vi "Open&Close Door Record.vi"(8 "error in (no error)":errorcluster, 11 "Para":T2={"url"="http://dev.watersystem.com.cn:36091", "AccessToken"="data&auXnb5fsZ6235te50ySpHm7Nhv4", "mn"="admin", "isOpenDoor"=FALSE}) -> (0 "error out":errorcluster, 3 "response":T1)   [LabVIEW 2016, in "opSignIn.lvlib"]
uses:
  <vilib>/httpClient/POSTBuffer.vi
  opSignIn.lvlib
  <vilib>/httpClient/LabVIEWHTTPClient.lvlib
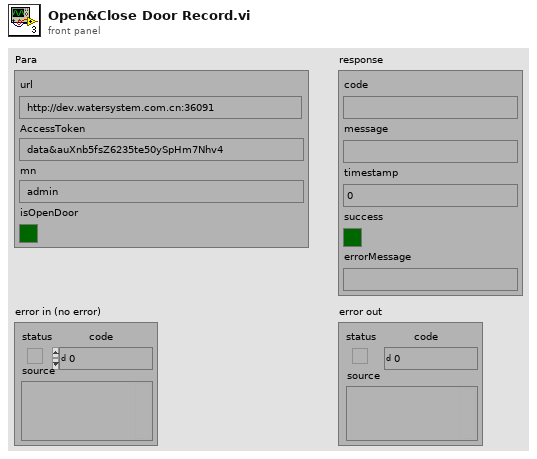
[diagram p1: front panel]
types:
  T1 = cluster{"code":string, "message":string, "timestamp":u64, "success":bool, "errorMessage":string}
  T2 = cluster{"url":string, "AccessToken":string, "mn":string, "isOpenDoor":bool}
  T3 = cluster{"code":string, "message":string, "timestamp":u64, "success":bool}
  T4 = typedef "LabVIEWHTTPClient.lvlib/ClientHandle.ctl" = refnum<k1>
  T5 = cluster{"code":string, "message":string, "timestamp":u64, "success":bool, string}
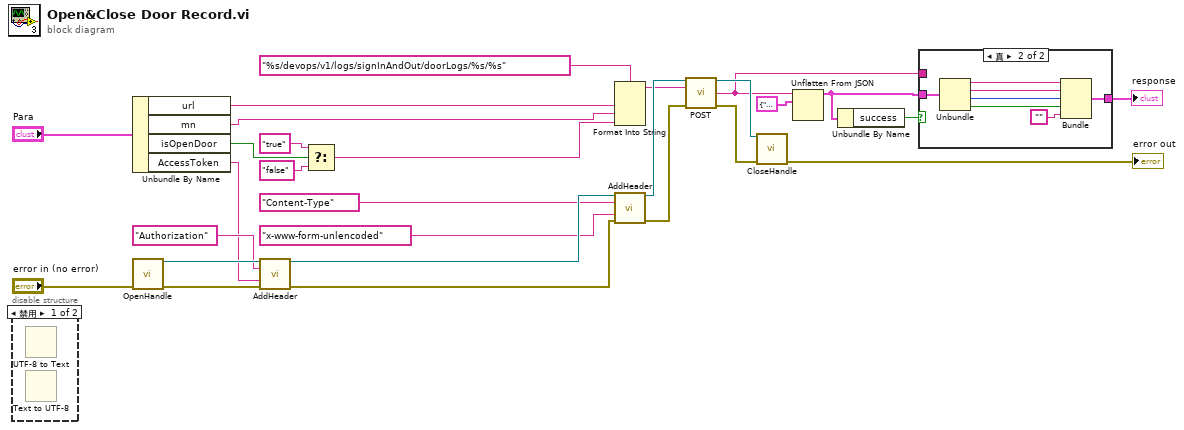
[diagram p0: block diagram]
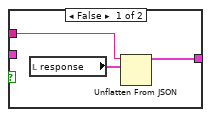
[diagram p2: hidden frame]
diagram:
  n1 = disable-structure shown="禁用" {
    frame Disabled {
      n2 = UTF-8 to Text() -> ()  [unwired: 3 in, 2 out]
      n3 = Text to UTF-8() -> ()  [unwired: 3 in, 2 out]
    }
    frame Enabled {
    }
  }
  n4 = Unbundle By Name("Para") -> ("url"=w6:string, "mn"=w9:string, "isOpenDoor"=w8:bool, "AccessToken"=w7:string)
  n5 = call <vilib>:"OpenHandle.vi"("error in (no error)"="error in (no error)") -> ("client handle out"=w28:T4, "error out"=w27:errorcluster)  [unwired: 13 in]
  n6 = call <vilib>:"AddHeader.vi"("client handle"=w28, "header"="Authorization", "value"=w7, "error in (no error)"=w27) -> ("client handle out"=w23:T4, "error out"=w22:errorcluster)  [unwired: 10 in]
  n7 = Select(t="true", s=w8, f="false") -> (s? t:f=w11:string)
  n8 = Format Into String(format string="%s/devops/v1/logs/signInAndOut/doorLogs/%s/%s" ("url"), w6, w9, w11) -> (resulting string=w14:string)  [unwired: 2 in, 1 out]
  n9 = call <vilib>:"AddHeader.vi"("client handle"=w23, "header"="Content-Type", "value"="x-www-form-unlencoded", "error in (no error)"=w22) -> ("client handle out"=w19:T4, "error out"=w18:errorcluster)  [unwired: 10 in]
  n10 = call-poly <vilib>:"POST.vi"("client handle"=w19, "url"=w14, "error in (no error)"=w18) -> ("client handle out"=w17:T4, "body"=w3:string, "error out"=w16:errorcluster)  [unwired: 9 in, 1 out]
  n11 = call <vilib>:"CloseHandle.vi"("client handle"=w17, "error in (no error)"=w16) -> ("error out"=→"error out":errorcluster)  [unwired: 13 in]
  n12 = Unflatten From JSON(JSON string=w3, type and defaults=T3 {"code"="", "message"="", "timestamp"=0, "success"=FALSE} ("response")) -> (value=w2:T3)  [unwired: 5 in, 1 out]
  n13 = Unbundle By Name(w2) -> ("success"=w5:bool)
  n14 = case shown="真" w5 {
    tunnel: [w30 w36] -> w4
    tunnel: w3 -> [w29 _]
    tunnel: w2 -> [_ w38]
    frame False {
      n15 = local read "response"() -> (w31:T1)
      n16 = Unflatten From JSON(JSON string=w29, type and defaults=w31) -> (value=w30:T1)  [unwired: 5 in, 1 out]
    }
    frame True {
      n17 = Unbundle(w38) -> ("code"=w37:string, "message"=w35:string, "timestamp"=w34:u64, "success"=w33:bool)
      n18 = Bundle("code"=w37, "message"=w35, "timestamp"=w34, "success"=w33, "") -> (w36:T5)  [unwired: 1 in]
    }
  }
  "response" <- w4
